vi "Get All Connections.vi"(8 "error in (no error)":errorcluster, 11 "Route Manager in":refnum<class "Route Manager.lvclass">) -> (0 "error out":errorcluster, 2 "connections":T1[](array[typedef]))   [LabVIEW 2015, in "Route Manager.lvclass"]
uses:
  Route Manager.lvclass
  Connection.ctl
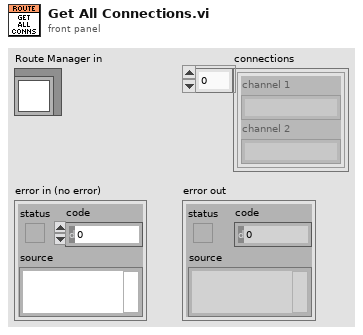
[diagram p1: front panel]
types:
  T1 = typedef "Route Manager.lvclass/Connection.ctl" = cluster{"channel 1":string, "channel 2":string}
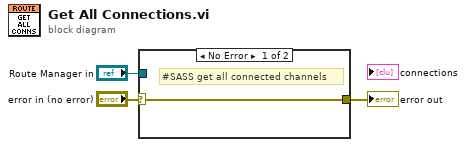
[diagram p0: block diagram]
diagram:
  n1 = case shown="No Error" "error in (no error)" {
    selector: "error in (no error)" -> [w4 w5]
    tunnel: [w4 w5] -> w2
    tunnel: "Route Manager in" -> [_ _]
    frame No Error {
      # "#SASS get all connected channels"
    }
    frame Error {
    }
  }
  "error out" <- w2
